vi "MTS_AutoLaserPower2.vi"(4 "Laser 1/3 ?":bool, 5 "Laser 1-2 ?":bool, 6 "Laser Power Callib":dbl=1.0, 7 "CAN Adress":u32, 9 "Step":dbl=20.0, 10 "Offset":dbl, 11 "N Points":i32=6) -> (0 "Error Setting Position":bool, 2 "Positions":dbl[](array[numeric]), 3 "Intensitys":dbl[](array[numeric]))   [LabVIEW 2013]
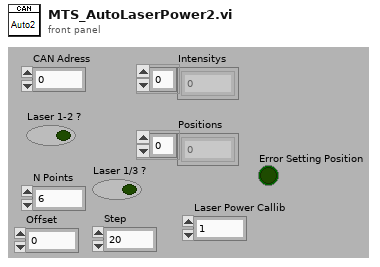
[diagram p1: front panel]
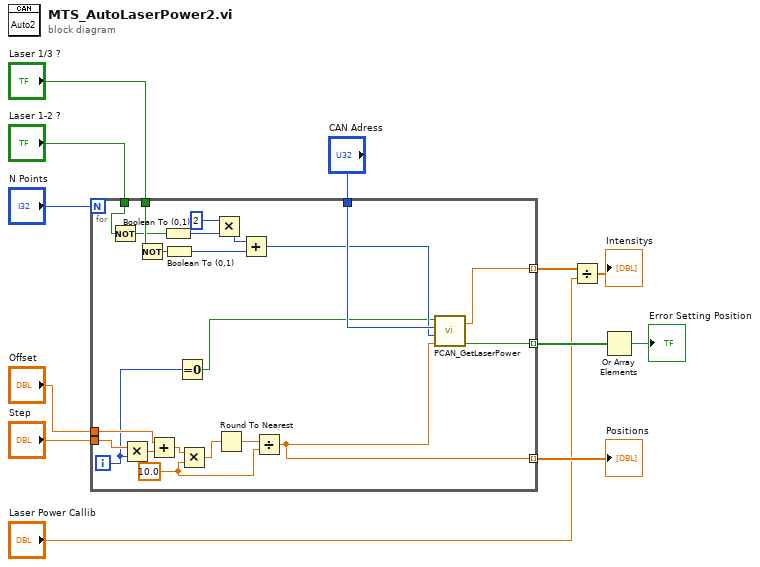
[diagram p0: block diagram]
diagram:
  n1 = for {
    N: "N Points" -> [_]
    tunnel: "CAN Adress" -> [w34]
    tunnel: "Laser 1-2 ?" -> [w16]
    tunnel: [w32] -> w3 mode=indexing
    tunnel: [w24] -> w12 mode=indexing
    tunnel: [w33] -> w8 mode=indexing
    tunnel: "Step" -> [w31]
    tunnel: "Offset" -> [w29]
    tunnel: "Laser 1/3 ?" -> [w19]
    i -> [w14]
    w25 = 10.0 ("y")
    n2 = Not(x=w16) -> (.not. x?=w17:bool)
    n3 = Multiply(x=w31, y=w14) -> (x*y=w30:dbl)
    n4 = Not(x=w19) -> (.not. x?=w18:bool)
    n5 = Add(x=w29, y=w30) -> (x+y=w28:dbl)
    n6 = Boolean To (0,1)(Boolean=w17) -> (0, 1=w23:i16)
    n7 = Boolean To (0,1)(Boolean=w18) -> (0, 1=w20:i16)
    n8 = Equal To 0?(x=w14) -> (x = 0?=w13:bool)
    n9 = Multiply(x=w28, y=w25) -> (x*y=w27:dbl)
    n10 = Multiply(x=i16 2, y=w23) -> (x*y=w21:i16)
    n11 = Round To Nearest(number=w27) -> (nearest integer value=w26:dbl)
    n12 = Add(x=w21, y=w20) -> (x+y=w15:i16)
    n13 = Divide(x=w26, y=w25) -> (x/y=w24:dbl)
    n14 = call "PCAN_GetLaserPower.vi"("Position"=w24, "Laser No"=w15, "CAN Adress"=w34, "Extra Wait"=w13) -> ("Error ?"=w33:bool, "Intensity (a.u.)"=w32:dbl)
  }
  "Positions" <- w12
  n15 = Divide(x=w3, y="Laser Power Callib") -> (x/y=→"Intensitys":dbl[])
  n16 = Or Array Elements(Boolean array=w8) -> (logical OR=→"Error Setting Position":bool)
